vi "niRFUtil WFM Invert Spectrum.vi"(1 "Spectrum Inverted":T1, 3 "Waveform In":T2 {"y" format="%.2f"; "dx" format="%^.2e"; "x0" format="%^.2e"}) -> (0 "Waveform Out":T2 {"y" format="%.2f"; "dx" format="%^.2e"; "x0" format="%^.2e"})   [LabVIEW 2015, in "niRFUtil.lvlib"]
uses:
  niRFUtil.lvlib
  Includes/niRFUtil INC Complex Waveform.ctl
  Includes/niRFUtil INC Complex Array.ctl
  Includes/niRFUtil INC Spectrum Inverted.ctl
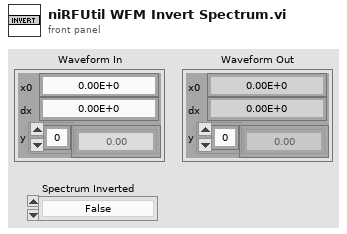
[diagram p1: front panel]
types:
  T1 = typedef "niRFUtil.lvlib/niRFUtil INC Spectrum Inverted.ctl" = enum16{"False", "True"}
  T2 = typedef "niRFUtil.lvlib/niRFUtil INC Complex Waveform.ctl" = cluster{"x0":dbl, "dx":dbl, "y":T3}
  T3 = typedef "niRFUtil.lvlib/niRFUtil INC Complex Array.ctl" = csg[]
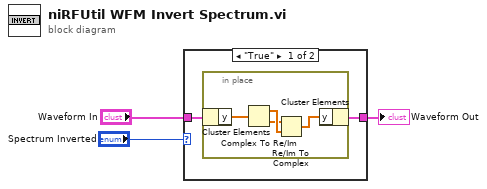
[diagram p0: block diagram]
diagram:
  n1 = case shown="\"True\"" "Spectrum Inverted" {
    tunnel: "Waveform In" -> [w5 w10]
    tunnel: [w4 w10] -> w2
    frame "True" {
      n2 = in-place {
        n3 = in-place-cluster #1(w5) -> ("y"=w7:T3)
        n4 = Complex To Re/Im(x + iy=w7) -> (x=w9:sgl[], y=w8:sgl[])
        n5 = Re/Im To Complex(1:w9, 2:w8) -> (0:w6:csg[])
        n6 = in-place-cluster #1("y"=w6) -> (w4:T2)
      }
    }
    frame "False", Default {
    }
  }
  "Waveform Out" <- w2
